vi "XIPIN_Serial_RapidIO_Gen2_4_0.vi"   [LabVIEW 2017]
doc: "The Xilinx v4.0 Serial RapidIO Gen 2 Solution consists of Physical, Buffer and Logical Layer cores designed to the RapidIO v2.2 spec. Reference designs and development scripts are provided to support development of a customized, fully compliant system.\n------------------------------------\n<b>Need License</b> : Yes\n<b>Interface</b> : AXI4 AXI4-Stream"
uses:
  <vilib>/rvi/XilinxIP/XIPIN_XNode/niFpgaXIPIN.xnode
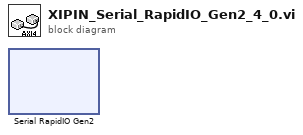
[diagram p0: block diagram]
diagram:
  n1 = xnode ("Serial RapidIO Gen2")() -> ()
